vi "T-Peak.vi"() -> ()   [LabVIEW 2013]
panel:
  in  "all rows":dbl[][](array[numeric])=[[19.8, 20.5, 21.3, 22.3, 23.3, 24.5, 25.6, 26.9, 28.1, 29.3], [100.0, 117.0, 200.0, 296.0, 392.0, 505.0, 615.0, 732.0, 863.0, 985.0]] format="%0.3f"
  out "Original Data Graph":cluster{"all rows":dbl[], "all rows":dbl[]}(graph)
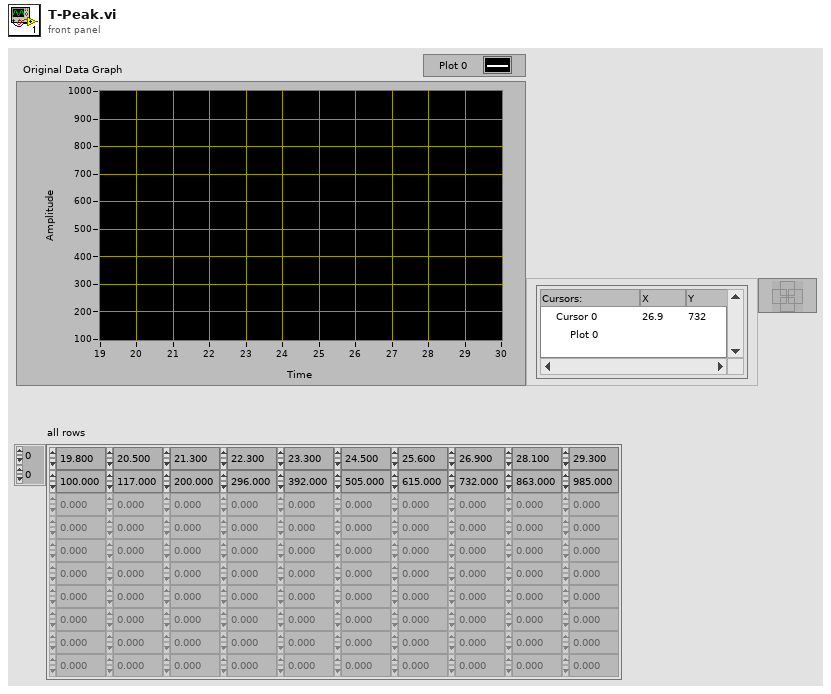
[diagram p1: front panel]
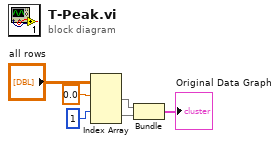
[diagram p0: block diagram]
diagram:
  n1 = Index Array(array="all rows", index (row) #1=0.0 ("index (row)"), index (row) #2=1 ("index (row)")) -> (element #1=w2:dbl[], element #2=w1:dbl[])  [unwired: 2 in]
  n2 = Bundle("all rows"=w2, "all rows"=w1) -> (→"Original Data Graph":cluster{"all rows":dbl[], "all rows":dbl[]})  [unwired: 1 in]
